vi "Zj(r,theta).vi"(4 "error in (no error)":errorcluster, 5 "theta":dbl, 6 "r":dbl, 7 "j (1)":i32=1) -> (0 "error out":errorcluster, 1 "m":i32, 2 "n":i32, 3 "Zj(r,theta)":dbl)   [LabVIEW 2012, in "Zernike Polynome.lvlib"]
doc: "This VI calculates Zj(r,theta)."
uses:
  Zernike Polynome.lvlib
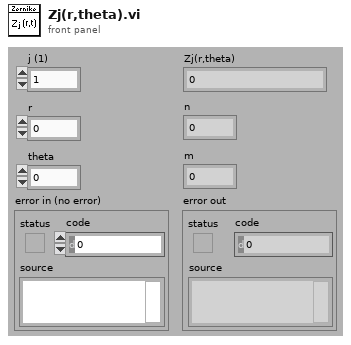
[diagram p1: front panel]
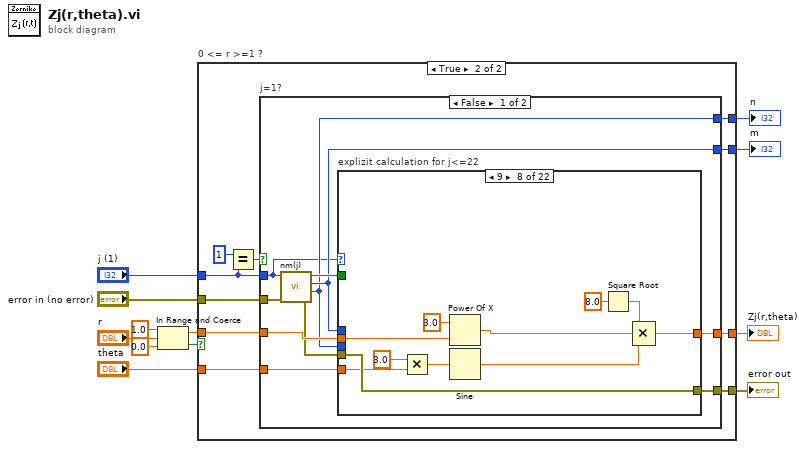
[diagram p0: block diagram]
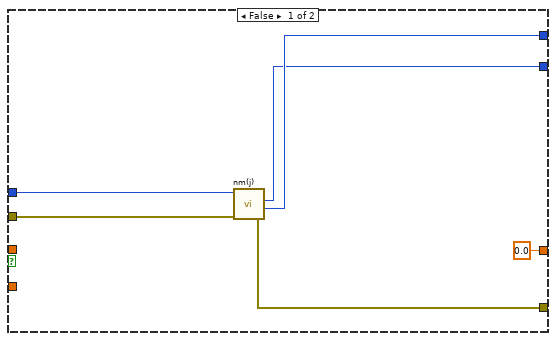
[diagram p2: hidden frame]
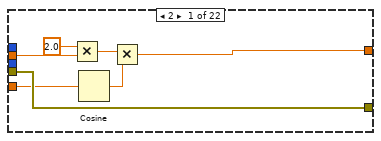
[diagram p3: hidden frame]
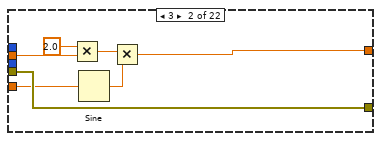
[diagram p4: hidden frame]
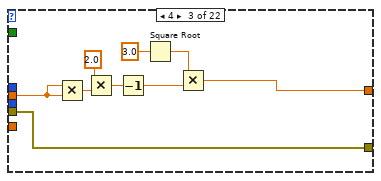
[diagram p5: hidden frame]
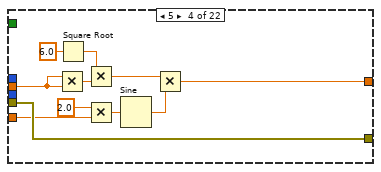
[diagram p6: hidden frame]
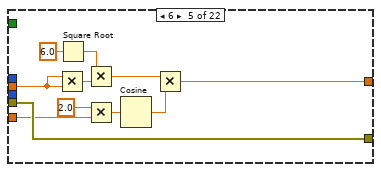
[diagram p7: hidden frame]
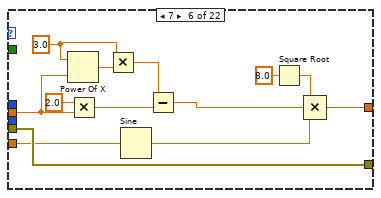
[diagram p8: hidden frame]
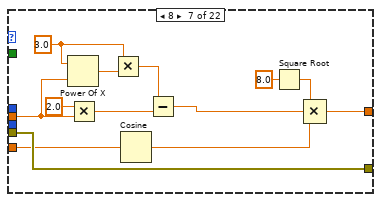
[diagram p9: hidden frame]
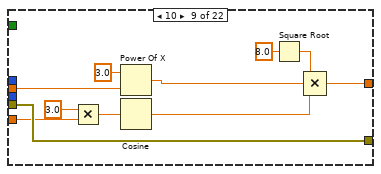
[diagram p10: hidden frame]
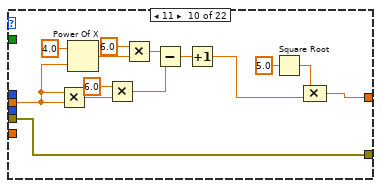
[diagram p11: hidden frame]
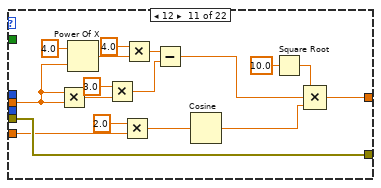
[diagram p12: hidden frame]
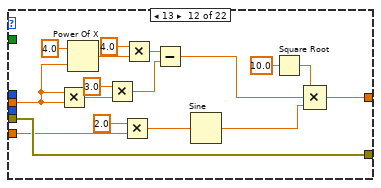
[diagram p13: hidden frame]
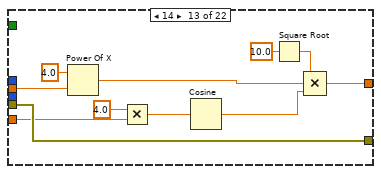
[diagram p14: hidden frame]
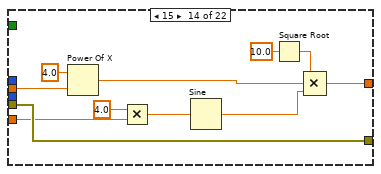
[diagram p15: hidden frame]
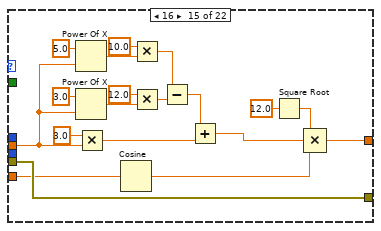
[diagram p16: hidden frame]
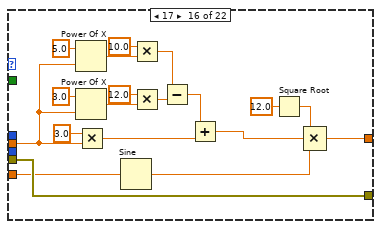
[diagram p17: hidden frame]
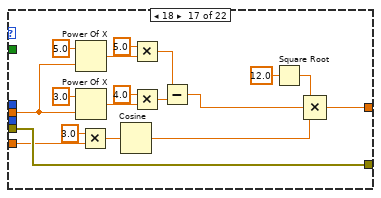
[diagram p18: hidden frame]
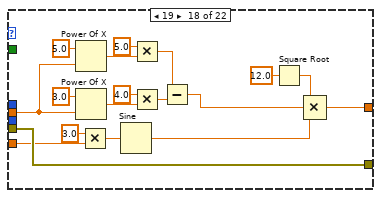
[diagram p19: hidden frame]
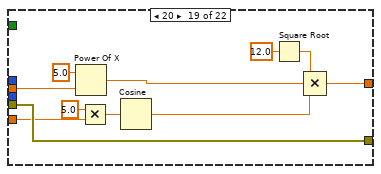
[diagram p20: hidden frame]
diagram:
  n1 = In Range and Coerce(upper limit=1.0, x="r", lower limit=0.0) -> (coerced(x)=w4:dbl, In Range?=w1:bool)
  n2 = case "0 <= r >=1 ?" shown="True" w1 {
    tunnel: "error in (no error)" -> [w17 w28]
    tunnel: [w16 w27] -> w11
    tunnel: [0.0 w26] -> w10
    tunnel: "j (1)" -> [w18 w24]
    tunnel: [w14 w22] -> w8
    tunnel: [w15 w21] -> w7
    tunnel: "theta" -> [_ w20]
    tunnel: w4 -> [_ w19]
    frame False {
      n3 = call "nm(j).vi"("error in (no error)"=w17, "j (1)"=w18) -> ("error out"=w16:errorcluster, "n"=w15:i32, "m"=w14:i32)  [unwired: 2 in, 1 out]
    }
    frame True {
      n4 = Equal?(x=1, y=w24) -> (x = y?=w25:bool)
      n5 = case "j=1?" shown="False" w25 {
        tunnel: w19 -> [w38 _]
        tunnel: w28 -> [w35 w354]
        tunnel: [w34 w354] -> w27
        tunnel: w24 -> [w30 _]
        tunnel: [w33 1.0] -> w26
        tunnel: [w32 w353] -> w22
        tunnel: [w31 w353] -> w21
        tunnel: w20 -> [w29 _]
        frame False {
          n6 = call "nm(j).vi"("error in (no error)"=w35, "j (1)"=w30) -> ("error out"=w36:errorcluster, "n"=w31:i32, "m"=w32:i32, "odd"=w37:bool)  [unwired: 2 in]
          n7 = case "explizit calculation for j<=22" shown="9" w30 {
            tunnel: w38 -> [w44 w51 w59 w71 w82 w93 w106 w117 w128 w138 w155 w172 w185 w196 w207 w226 w246 w264 w281 w292 w303 w326]
            tunnel: w37 -> [_ _ _ _ _ _ _ _ _ _ _ _ _ _ _ _ _ _ _ _ _ w325]
            tunnel: w36 -> [w45 w52 w61 w72 w83 w96 w109 w120 w131 w145 w162 w179 w190 w201 w220 w239 w257 w275 w286 w297 w316 w324]
            tunnel: [w45 w52 w61 w72 w83 w96 w109 w120 w131 w145 w162 w179 w190 w201 w220 w239 w257 w275 w286 w297 w316 w321] -> w34
            tunnel: [w39 w46 w54 w62 w73 w86 w100 w114 w125 w142 w159 w176 w187 w198 w214 w233 w253 w271 w282 w293 w313 w320] -> w33
            tunnel: w32 -> [_ _ _ _ _ _ _ _ _ _ _ _ _ _ _ _ _ _ _ _ _ w319]
            tunnel: w31 -> [_ _ _ _ _ _ _ _ _ _ _ _ _ _ _ _ _ _ _ _ _ w318]
            tunnel: w29 -> [w42 w49 _ w67 w78 w94 w107 w112 w123 _ w149 w166 w184 w195 w218 w237 w242 w260 w279 w290 _ w317]
            frame 2 {
              n8 = Multiply(x=2.0, y=w44) -> (x*y=w41:dbl)
              n9 = Cosine(x=w42) -> (cos(x)=w40:dbl)
              n10 = Multiply(x=w41, y=w40) -> (x*y=w39:dbl)
            }
            frame 3 {
              n11 = Multiply(x=2.0, y=w51) -> (x*y=w48:dbl)
              n12 = Sine(x=w49) -> (sin(x)=w47:dbl)
              n13 = Multiply(x=w48, y=w47) -> (x*y=w46:dbl)
            }
            frame 4 {
              n14 = Multiply(x=w59, y=w59) -> (x*y=w58:dbl)
              n15 = Multiply(x=2.0, y=w58) -> (x*y=w57:dbl)
              n16 = Decrement(x=w57) -> (x-1=w55:dbl)
              n17 = Square Root(x=3.0) -> (sqrt(x)=w53:dbl)
              n18 = Multiply(x=w53, y=w55) -> (x*y=w54:dbl)
            }
            frame 5 {
              n19 = Multiply(x=w71, y=w71) -> (x*y=w70:dbl)
              n20 = Square Root(x=6.0) -> (sqrt(x)=w68:dbl)
              n21 = Multiply(x=w68, y=w70) -> (x*y=w64:dbl)
              n22 = Multiply(x=2.0, y=w67) -> (x*y=w65:dbl)
              n23 = Sine(x=w65) -> (sin(x)=w63:dbl)
              n24 = Multiply(x=w64, y=w63) -> (x*y=w62:dbl)
            }
            frame 6 {
              n25 = Multiply(x=w82, y=w82) -> (x*y=w81:dbl)
              n26 = Square Root(x=6.0) -> (sqrt(x)=w79:dbl)
              n27 = Multiply(x=w79, y=w81) -> (x*y=w75:dbl)
              n28 = Multiply(x=2.0, y=w78) -> (x*y=w76:dbl)
              n29 = Cosine(x=w76) -> (cos(x)=w74:dbl)
              n30 = Multiply(x=w75, y=w74) -> (x*y=w73:dbl)
            }
            frame 7 {
              w84 = 3.0 ("y")
              n31 = Power Of X(1:w93, 2:w84) -> (0:w91:dbl)
              n32 = Multiply(x=2.0, y=w93) -> (x*y=w90:dbl)
              n33 = Multiply(x=w84, y=w91) -> (x*y=w85:dbl)
              n34 = Sine(x=w94) -> (sin(x)=w87:dbl)
              n35 = Subtract(x=w85, y=w90) -> (x-y=w88:dbl)
              n36 = Square Root(x=8.0) -> (sqrt(x)=w89:dbl)
              n37 = Compound Arithmetic op=MULTIPLY(w89, w88, w87) -> (w86:dbl)
            }
            frame 8 {
              w97 = 3.0 ("y")
              n38 = Power Of X(1:w106, 2:w97) -> (0:w98:dbl)
              n39 = Multiply(x=2.0, y=w106) -> (x*y=w104:dbl)
              n40 = Multiply(x=w97, y=w98) -> (x*y=w99:dbl)
              n41 = Cosine(x=w107) -> (cos(x)=w101:dbl)
              n42 = Subtract(x=w99, y=w104) -> (x-y=w102:dbl)
              n43 = Square Root(x=8.0) -> (sqrt(x)=w103:dbl)
              n44 = Compound Arithmetic op=MULTIPLY(w103, w102, w101) -> (w100:dbl)
            }
            frame 9 {
              n45 = Multiply(x=3.0, y=w112) -> (x*y=w111:dbl)
              n46 = Power Of X(1:w117, 2:3.0 ("y")) -> (0:w113:dbl)
              n47 = Sine(x=w111) -> (sin(x)=w115:dbl)
              n48 = Square Root(x=8.0) -> (sqrt(x)=w116:dbl)
              n49 = Compound Arithmetic op=MULTIPLY(w116, w113, w115) -> (w114:dbl)
            }
            frame 10 {
              n50 = Multiply(x=3.0, y=w123) -> (x*y=w122:dbl)
              n51 = Power Of X(1:w128, 2:3.0 ("y")) -> (0:w124:dbl)
              n52 = Cosine(x=w122) -> (cos(x)=w126:dbl)
              n53 = Square Root(x=8.0) -> (sqrt(x)=w127:dbl)
              n54 = Compound Arithmetic op=MULTIPLY(w127, w124, w126) -> (w125:dbl)
            }
            frame 11 {
              n55 = Multiply(x=w138, y=w138) -> (x*y=w136:dbl)
              n56 = Power Of X(1:w138, 2:4.0 ("y")) -> (0:w140:dbl)
              n57 = Multiply(x=6.0, y=w136) -> (x*y=w134:dbl)
              n58 = Multiply(x=6.0, y=w140) -> (x*y=w135:dbl)
              n59 = Subtract(x=w135, y=w134) -> (x-y=w133:dbl)
              n60 = Increment(x=w133) -> (x+1=w132:dbl)
              n61 = Square Root(x=5.0) -> (sqrt(x)=w143:dbl)
              n62 = Compound Arithmetic op=MULTIPLY(w143, w132) -> (w142:dbl)
            }
            frame 12 {
              n63 = Multiply(x=w155, y=w155) -> (x*y=w153:dbl)
              n64 = Power Of X(1:w155, 2:4.0 ("y")) -> (0:w157:dbl)
              n65 = Multiply(x=3.0, y=w153) -> (x*y=w150:dbl)
              n66 = Multiply(x=2.0, y=w149) -> (x*y=w147:dbl)
              n67 = Multiply(x=4.0, y=w157) -> (x*y=w152:dbl)
              n68 = Subtract(x=w152, y=w150) -> (x-y=w151:dbl)
              n69 = Cosine(x=w147) -> (cos(x)=w146:dbl)
              n70 = Square Root(x=10.0) -> (sqrt(x)=w160:dbl)
              n71 = Compound Arithmetic op=MULTIPLY(w160, w151, w146) -> (w159:dbl)
            }
            frame 13 {
              n72 = Multiply(x=w172, y=w172) -> (x*y=w170:dbl)
              n73 = Power Of X(1:w172, 2:4.0 ("y")) -> (0:w174:dbl)
              n74 = Multiply(x=3.0, y=w170) -> (x*y=w167:dbl)
              n75 = Multiply(x=2.0, y=w166) -> (x*y=w164:dbl)
              n76 = Multiply(x=4.0, y=w174) -> (x*y=w169:dbl)
              n77 = Subtract(x=w169, y=w167) -> (x-y=w168:dbl)
              n78 = Sine(x=w164) -> (sin(x)=w163:dbl)
              n79 = Square Root(x=10.0) -> (sqrt(x)=w177:dbl)
              n80 = Compound Arithmetic op=MULTIPLY(w177, w168, w163) -> (w176:dbl)
            }
            frame 14 {
              n81 = Power Of X(1:w185, 2:4.0 ("y")) -> (0:w180:dbl)
              n82 = Multiply(x=4.0, y=w184) -> (x*y=w182:dbl)
              n83 = Cosine(x=w182) -> (cos(x)=w181:dbl)
              n84 = Square Root(x=10.0) -> (sqrt(x)=w188:dbl)
              n85 = Compound Arithmetic op=MULTIPLY(w188, w180, w181) -> (w187:dbl)
            }
            frame 15 {
              n86 = Power Of X(1:w196, 2:4.0 ("y")) -> (0:w191:dbl)
              n87 = Multiply(x=4.0, y=w195) -> (x*y=w193:dbl)
              n88 = Sine(x=w193) -> (sin(x)=w192:dbl)
              n89 = Square Root(x=10.0) -> (sqrt(x)=w199:dbl)
              n90 = Compound Arithmetic op=MULTIPLY(w199, w191, w192) -> (w198:dbl)
            }
            frame 16 {
              n91 = Power Of X(1:w207, 2:5.0 ("y")) -> (0:w212:dbl)
              n92 = Power Of X(1:w207, 2:3.0 ("y")) -> (0:w208:dbl)
              n93 = Multiply(x=3.0, y=w207) -> (x*y=w205:dbl)
              n94 = Cosine(x=w218) -> (cos(x)=w215:dbl)
              n95 = Multiply(x=10.0, y=w212) -> (x*y=w213:dbl)
              n96 = Multiply(x=12.0, y=w208) -> (x*y=w206:dbl)
              n97 = Subtract(x=w213, y=w206) -> (x-y=w204:dbl)
              n98 = Add(x=w204, y=w205) -> (x+y=w203:dbl)
              n99 = Square Root(x=12.0) -> (sqrt(x)=w216:dbl)
              n100 = Compound Arithmetic op=MULTIPLY(w216, w203, w215) -> (w214:dbl)
            }
            frame 17 {
              n101 = Power Of X(1:w226, 2:5.0 ("y")) -> (0:w231:dbl)
              n102 = Power Of X(1:w226, 2:3.0 ("y")) -> (0:w227:dbl)
              n103 = Multiply(x=3.0, y=w226) -> (x*y=w224:dbl)
              n104 = Sine(x=w237) -> (sin(x)=w234:dbl)
              n105 = Multiply(x=10.0, y=w231) -> (x*y=w232:dbl)
              n106 = Multiply(x=12.0, y=w227) -> (x*y=w225:dbl)
              n107 = Subtract(x=w232, y=w225) -> (x-y=w223:dbl)
              n108 = Add(x=w223, y=w224) -> (x+y=w222:dbl)
              n109 = Square Root(x=12.0) -> (sqrt(x)=w235:dbl)
              n110 = Compound Arithmetic op=MULTIPLY(w235, w222, w234) -> (w233:dbl)
            }
            frame 18 {
              n111 = Power Of X(1:w246, 2:5.0 ("y")) -> (0:w251:dbl)
              n112 = Power Of X(1:w246, 2:3.0 ("y")) -> (0:w247:dbl)
              n113 = Multiply(x=3.0, y=w242) -> (x*y=w241:dbl)
              n114 = Cosine(x=w241) -> (cos(x)=w254:dbl)
              n115 = Multiply(x=5.0, y=w251) -> (x*y=w252:dbl)
              n116 = Multiply(x=4.0, y=w247) -> (x*y=w245:dbl)
              n117 = Subtract(x=w252, y=w245) -> (x-y=w244:dbl)
              n118 = Square Root(x=12.0) -> (sqrt(x)=w255:dbl)
              n119 = Compound Arithmetic op=MULTIPLY(w255, w244, w254) -> (w253:dbl)
            }
            frame 19 {
              n120 = Power Of X(1:w264, 2:5.0 ("y")) -> (0:w269:dbl)
              n121 = Power Of X(1:w264, 2:3.0 ("y")) -> (0:w265:dbl)
              n122 = Multiply(x=3.0, y=w260) -> (x*y=w259:dbl)
              n123 = Sine(x=w259) -> (sin(x)=w272:dbl)
              n124 = Multiply(x=5.0, y=w269) -> (x*y=w270:dbl)
              n125 = Multiply(x=4.0, y=w265) -> (x*y=w263:dbl)
              n126 = Subtract(x=w270, y=w263) -> (x-y=w262:dbl)
              n127 = Square Root(x=12.0) -> (sqrt(x)=w273:dbl)
              n128 = Compound Arithmetic op=MULTIPLY(w273, w262, w272) -> (w271:dbl)
            }
            frame 20 {
              n129 = Power Of X(1:w281, 2:5.0 ("y")) -> (0:w276:dbl)
              n130 = Multiply(x=5.0, y=w279) -> (x*y=w278:dbl)
              n131 = Cosine(x=w278) -> (cos(x)=w283:dbl)
              n132 = Square Root(x=12.0) -> (sqrt(x)=w284:dbl)
              n133 = Compound Arithmetic op=MULTIPLY(w284, w276, w283) -> (w282:dbl)
            }
            frame 21 {
              n134 = Power Of X(1:w292, 2:5.0 ("y")) -> (0:w287:dbl)
              n135 = Multiply(x=5.0, y=w290) -> (x*y=w289:dbl)
              n136 = Sine(x=w289) -> (sin(x)=w294:dbl)
              n137 = Square Root(x=12.0) -> (sqrt(x)=w295:dbl)
              n138 = Compound Arithmetic op=MULTIPLY(w295, w287, w294) -> (w293:dbl)
            }
            frame 22 {
              n139 = Multiply(x=w303, y=w303) -> (x*y=w308:dbl)
              n140 = Power Of X(1:w303, 2:6.0 ("y")) -> (0:w305:dbl)
              n141 = Power Of X(1:w303, 2:4.0 ("y")) -> (0:w311:dbl)
              n142 = Multiply(x=12.0, y=w308) -> (x*y=w299:dbl)
              n143 = Multiply(x=20.0, y=w305) -> (x*y=w302:dbl)
              n144 = Multiply(x=30.0, y=w311) -> (x*y=w301:dbl)
              n145 = Subtract(x=w302, y=w301) -> (x-y=w300:dbl)
              n146 = Add(x=w300, y=w299) -> (x+y=w298:dbl)
              n147 = Decrement(x=w298) -> (x-1=w307:dbl)
              n148 = Square Root(x=7.0) -> (sqrt(x)=w314:dbl)
              n149 = Compound Arithmetic op=MULTIPLY(w314, w307) -> (w313:dbl)
            }
            frame Default {
              n150 = call "Rnm(r).vi"("error in (no error)"=w324, "n"=w318, "r"=w326, "m"=w319) -> ("error out"=w322:errorcluster, "R nm (r)"=w323:dbl)  [unwired: 2 in]
              n151 = case shown="No Error" w322 {
                selector: w322 -> [w330 w352]
                tunnel: w325 -> [w335 _]
                tunnel: w319 -> [w334 _]
                tunnel: w318 -> [w333 _]
                tunnel: w323 -> [w331 _]
                tunnel: [w330 w352] -> w321
                tunnel: [w329 0.0] -> w320
                tunnel: w317 -> [w327 _]
                frame No Error {
                  n152 = Increment(x=w333) -> (x+1=w328:i32)
                  n153 = Square Root(x=w328) -> (sqrt(x)=w332:dbl)
                  n154 = Multiply(x=w332, y=w331) -> (x*y=w336:dbl)
                  n155 = case "m?" shown="Default" w334 {
                    selector: w334 -> [w343 _]
                    tunnel: w336 -> [w341 w350]
                    tunnel: [w338 w350] -> w329
                    tunnel: w335 -> [w344 _]
                    tunnel: w327 -> [w337 _]
                    frame Default {
                      n156 = Multiply(x=w343, y=w337) -> (x*y=w345:dbl)
                      n157 = case "True: odd" shown="False" w344 {
                        tunnel: w345 -> [w347 w348]
                        tunnel: [w346 w349] -> w342
                        frame False {
                          n158 = Cosine(x=w347) -> (cos(x)=w346:dbl)
                        }
                        frame True {
                          n159 = Sine(x=w348) -> (sin(x)=w349:dbl)
                        }
                      }
                      n160 = Square Root(x=2.0) -> (sqrt(x)=w339:dbl)
                      n161 = Compound Arithmetic op=MULTIPLY(w342, w341, w339) -> (w338:dbl)
                    }
                    frame 0 {
                    }
                  }
                }
                frame Error {
                }
              }
            }
          }
        }
        frame True {
          w353 = 0 ("n")
        }
      }
    }
  }
  "error out" <- w11
  "Zj(r,theta)" <- w10
  "m" <- w8
  "n" <- w7
